vi "Problem 6.vi"() -> ()   [LabVIEW 2025]
panel:
  out "Difference between the sum of the squares of the first 100 natural numbers and the square of the sum":i32
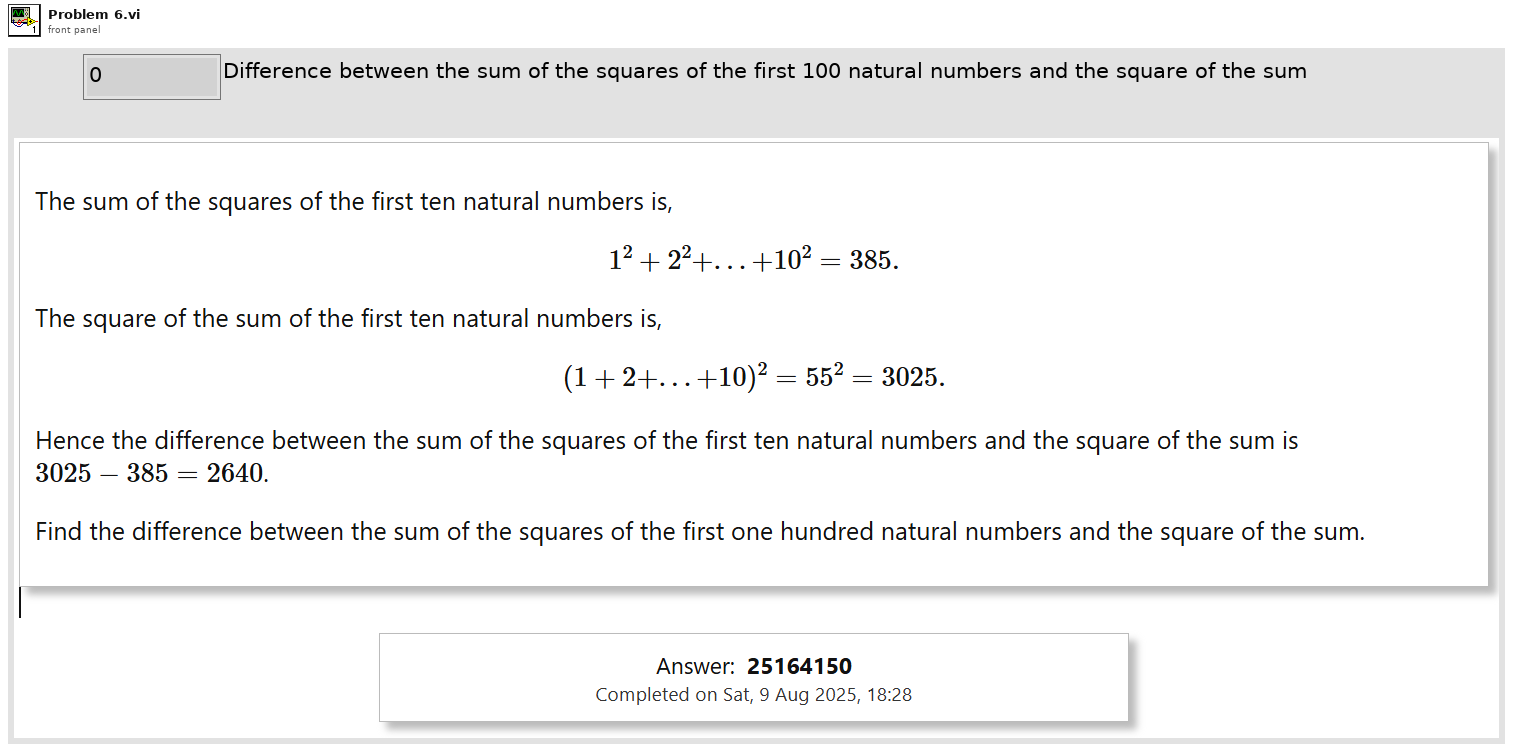
[diagram p1: front panel]
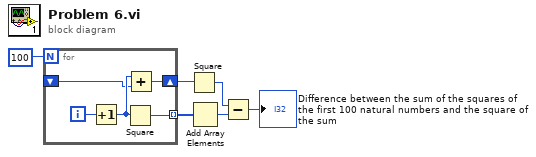
[diagram p0: block diagram]
diagram:
  n1 = for {
    N: 100 -> [_]
    tunnel: [w11] -> w5 mode=indexing
    shift-right: [w8] -> w4
    shift-left: _ -> [w7]
    i -> [w10]
    n2 = Increment(x=w10) -> (x+1=w9:i32)
    n3 = Square(x=w9) -> (x^2=w11:i32)
    n4 = Add(x=w9, y=w7) -> (x+y=w8:i32)
  }
  n5 = Square(x=w4) -> (x^2=w3:i32)
  n6 = Add Array Elements(numeric array=w5) -> (sum=w2:i32)
  n7 = Subtract(x=w3, y=w2) -> (x-y=→"Difference between the sum of the squares of the first 100 natural numbers and the square of the sum":i32)
